vi "读取2601B.vi"(8 "error in (no error)":errorcluster caption="错误输入（无错误）", 11 "2601B输入":refnum<class "2601B.lvclass">) -> (0 "error out":errorcluster caption="错误输出", 2 "2601B":refnum<visa-resource-name>, 3 "2601B输出":refnum<class "2601B.lvclass">)   [LabVIEW 2020, in "2601B.lvclass"]
uses:
  2601B.lvclass
  2601B.lvclass/2601B.ctl
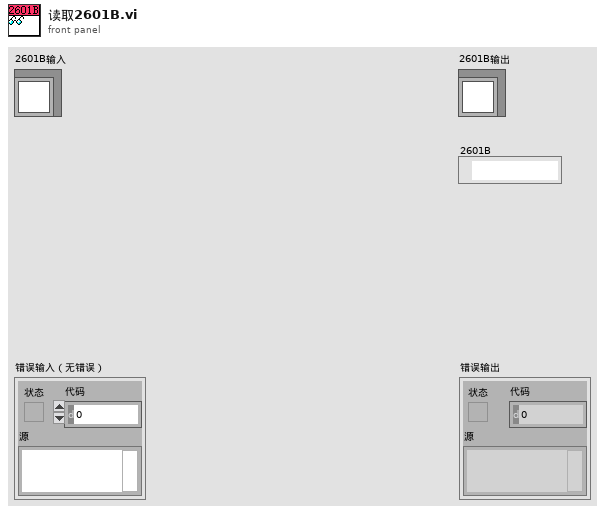
[diagram p1: front panel]
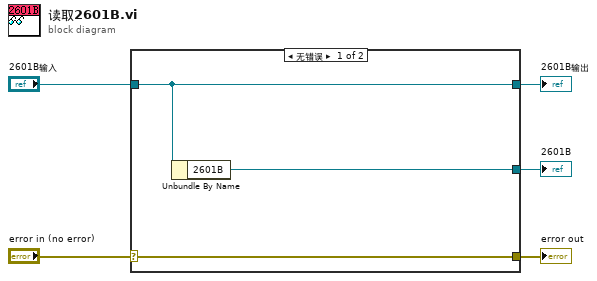
[diagram p0: block diagram]
diagram:
  n1 = case shown="无错误" "error in (no error)" {
    selector: "error in (no error)" -> [w8 w9]
    tunnel: [w8 w9] -> w4
    tunnel: [w7 w10] -> w2
    tunnel: "2601B输入" -> [w7 w10]
    tunnel: [w6 _] -> w1
    frame No Error {
      n2 = Unbundle By Name(w7) -> ("2601B"=w6:refnum<visa-resource-name>)
    }
    frame Error {
    }
  }
  "error out" <- w4
  "2601B输出" <- w2
  "2601B" <- w1
